vi "GaussianPeakFinder.vi"(3 "Mode":T4, 5 "Traverse line In":T1 {"Carrier_2 Q (l/min)" format="%#.2f"; "Row Duration (mins)" format="%#.1f"; "Row No" min=0; "Trace Gas Concentration (%)" min=0.0 format="%#_4f"; "Carrier_1 Q (l/min)" format="%#.2f"; "Tunnel Speed" format="%#.2f"; "Start X" format="%#.2f"; "Start Y" format="%#.2f"; "Start Z" format="%#.2f"; "End X" format="%#.2f"; "End Y" format="%#.2f"; "End Z" format="%#.2f"; "Averaging time (min)" min=0.0 format="%#.2f"}) -> (0 "Error Message":string, 1 "Status":T5, 2 "Traverse line Out":T1 {"Carrier_2 Q (l/min)" format="%#.2f"; "Row Duration (mins)" format="%#.1f"; "Row No" min=0; "Trace Gas Concentration (%)" min=0.0 format="%#_4f"; "Carrier_1 Q (l/min)" format="%#.2f"; "Tunnel Speed" format="%#.2f"; "Start X" format="%#.2f"; "Start Y" format="%#.2f"; "Start Z" format="%#.2f"; "End X" format="%#.2f"; "End Y" format="%#.2f"; "End Z" format="%#.2f"; "Averaging time (min)" min=0.0 format="%#.2f"})   [LabVIEW 2015]
uses:
  Gen Trav/Traverse_cluster.ctl
  Gen Trav/Spacing.ctl
  Controls/Multi_run_mode.ctl
  Controls/User_Specific_mode.ctl
  Gen Trav/Multi_Run_Status.ctl
  Controls/Setup.ctl
  Controls/Save_Data.ctl
  Utilities/gaussianFit/GaussianGlobal.vi
panel:
  in  "Tab Control":enum32{"GaussianFitGraph", "RunVINamed"}(tab)
  in  "nPointsInRake":i32=3
  out "nPointsSampled":i32
  in  "SpreadFactor":dbl=0.8
  in  "Turbulence":dbl=0.2
  in  "SampleLengthMultiplier":dbl=2.5
  out "MeasurementCenter":sgl
  # "X           Y            Z"
  # "Start"
  # "End"
  # "X           Y            Z"
  # "Start"
  # "End"
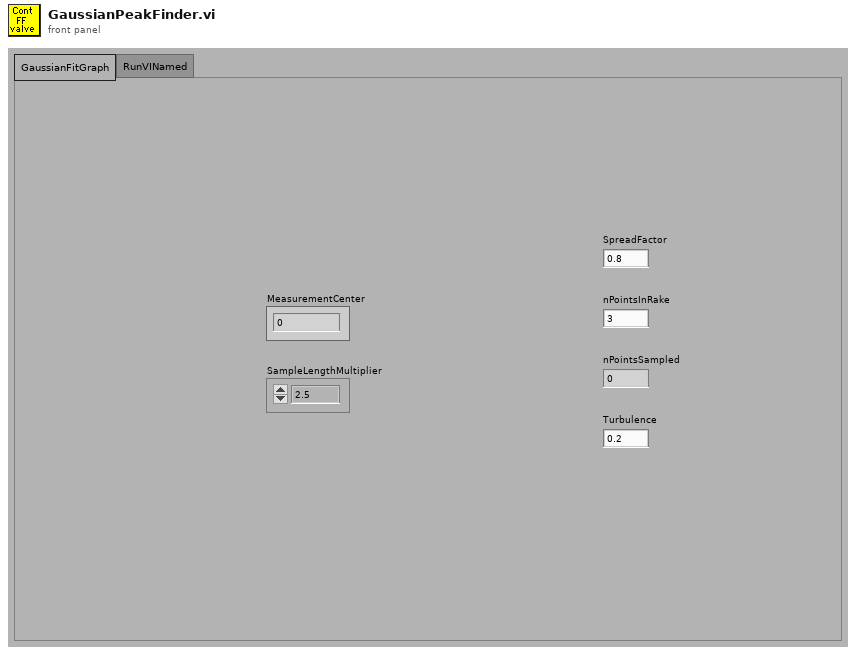
[diagram p1: front panel]
types:
  T1 = typedef "Traverse_cluster.ctl" = cluster{"Start X":sgl, "Start Y":sgl, "Start Z":sgl, "End X":sgl, "End Y":sgl, "End Z":sgl, "No. of pts.":i32, "Spacing":T2, "Filename":path, "Tunnel Speed":dbl, "Averaging time (min)":dbl, "Extra Commands":string, "Carrier_1 Q (l/min)":dbl, "Carrier_2 Q (l/min)":dbl, "Trace Gas Concentration (%)":dbl, "Specific Arguments":string, "Comments":string, "Row No":i32, "Row Type Selector":T3, "Completion time":string, "Row Duration (mins)":dbl, "No. of Valid pts.":i32, "Meas Setup File":string}
  T2 = typedef "Spacing.ctl" = enum16{"Linear", "Log", "Gauss", "Specified", "N/A"}
  T3 = typedef "Multi_run_mode.ctl" = enum16{"Move Traverse Only", "Set Tunnel Speed Only", "Set Source Only", "Set Measurement Conditions", "Single Measurement", "Vertical Profile", "Lateral Profile", "Longitudinal Profile", "Explore Volume", "Multi-Axis Profile", "Auto Calibrate", "Meas Fast FID Bkgnd", "Check Beam Power", "Scanning Valve Measurement", "Run VI Named:", "Set ADAM Ch", "Wait (minutes)", "Send Message", "Synchronize With:", "Fall Back to this Row", "Turn Off Row Repeating", "Blank Row", "Traverse 3D Volume"}
  T4 = typedef "User_Specific_mode.ctl" = enum16{"Check VI only", "Run VI"}
  T5 = typedef "Multi_Run_Status.ctl" = enum16{"Continue", "Jump to Next Point", "Jump to Next Row", "Jump To Fall Back", "Terminate Run"}
  T6 = typedef "Save_Data.ctl" = enum16{"Save No Data", "Save Data"}
  T7 = typedef "Setup.ctl" = enum16{"Run Program", "Show Setup", "Save Current Setup", "Setup Front Panel"}
  T8 = typedef "Status_Cluster.ctl" = cluster{"Status":T5, "Error Type":string, "Error Description":string}
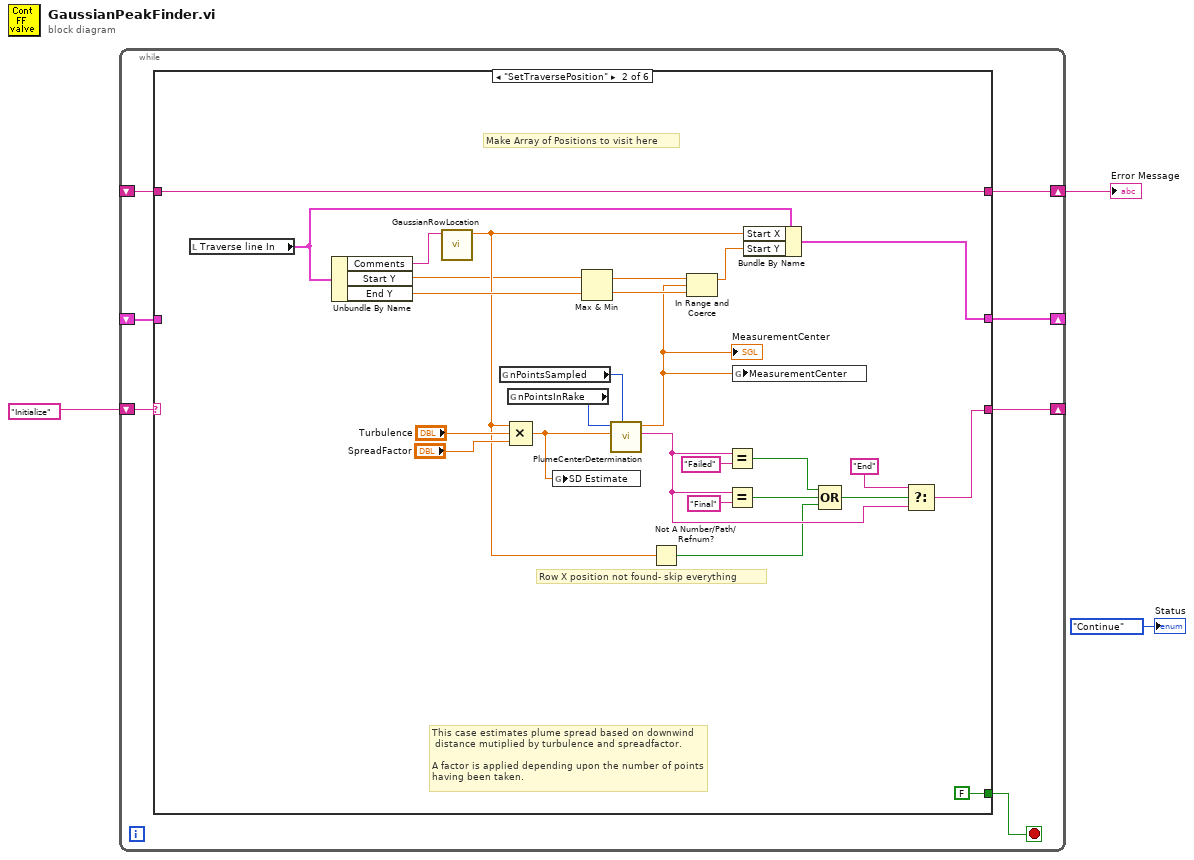
[diagram p0: block diagram]
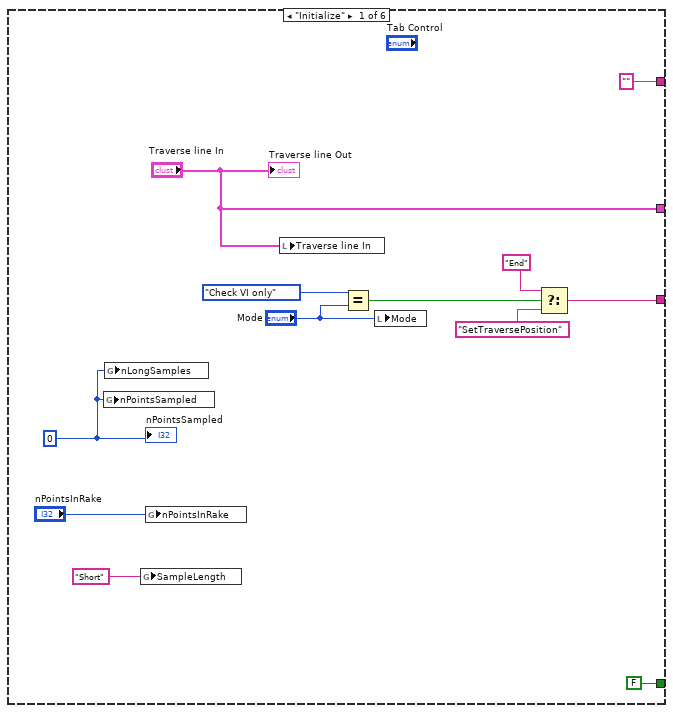
[diagram p2: hidden frame]
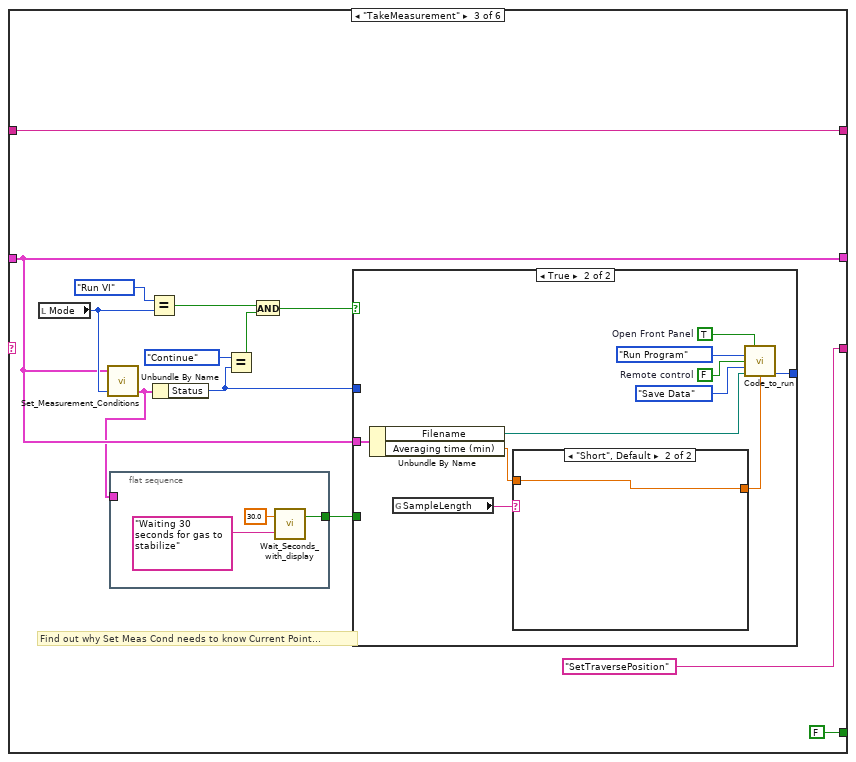
[diagram p3: hidden frame]
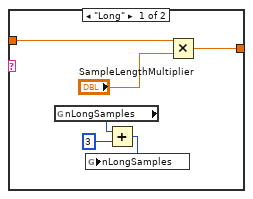
[diagram p5: hidden frame]
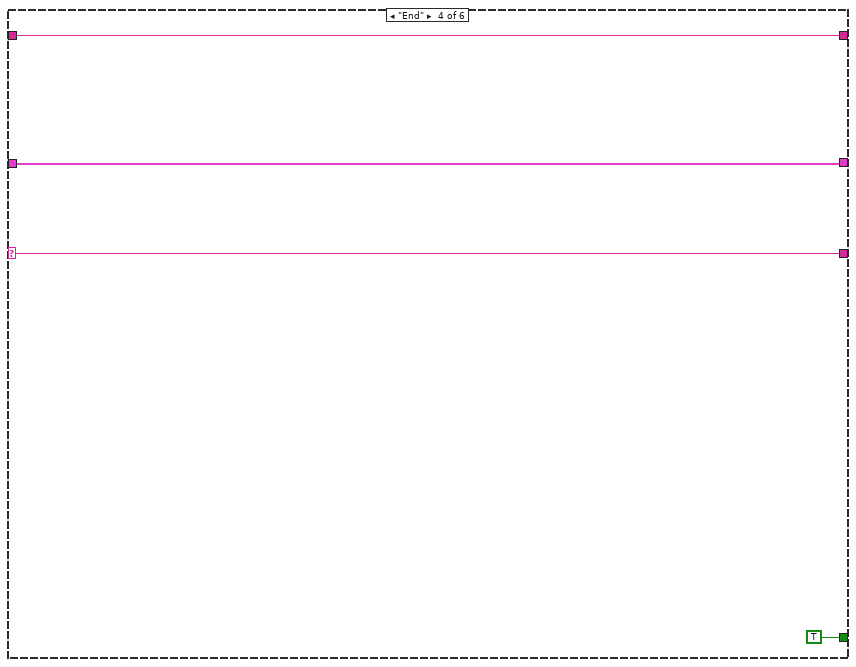
[diagram p6: hidden frame]
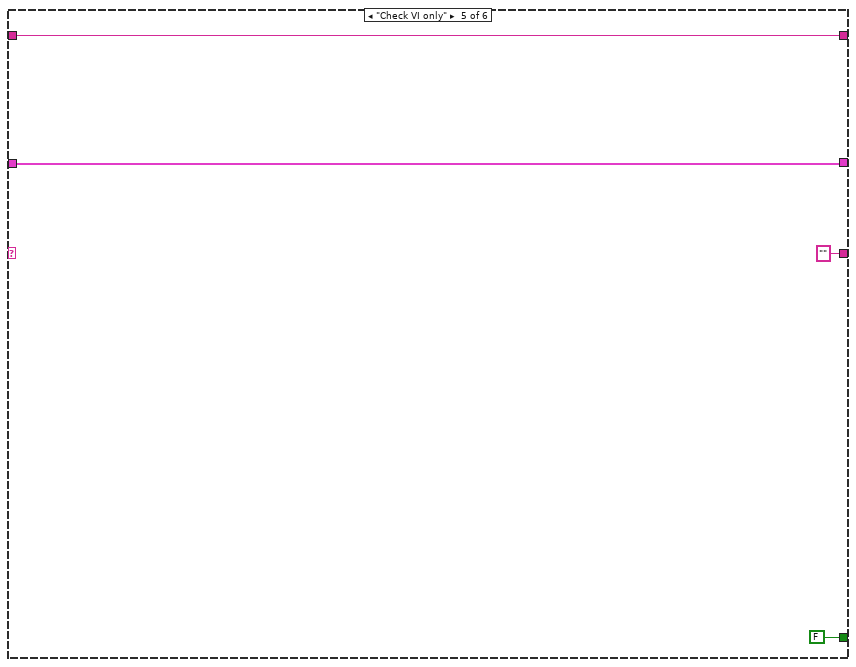
[diagram p7: hidden frame]
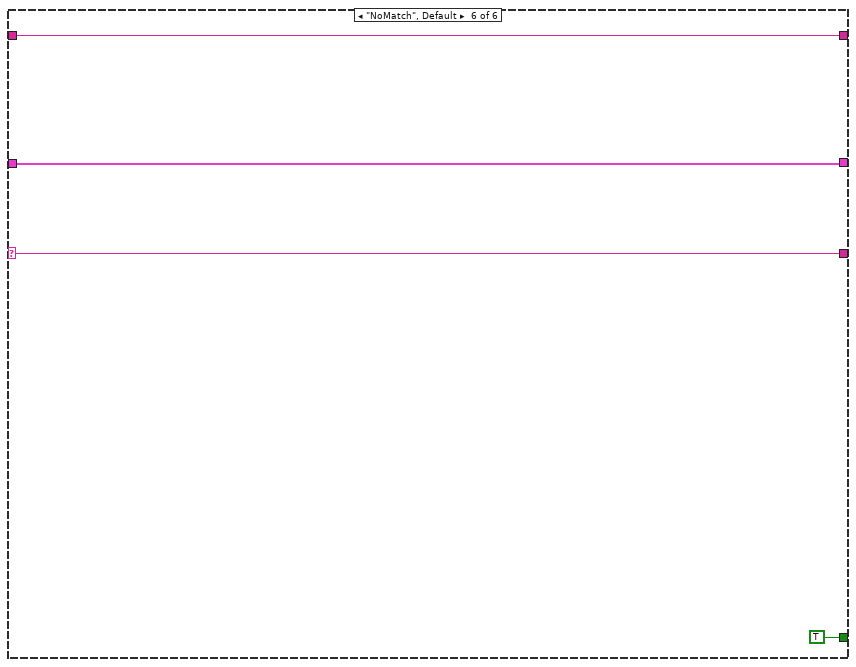
[diagram p8: hidden frame]
diagram:
  n1 = while {
    shift-right: [w8] -> _
    shift-left: _ -> [w7]
    shift-right: [w10] -> w2
    shift-left: _ -> [w5]
    shift-right: [w4] -> _
    shift-left: "Initialize" -> [w9]
    stop <- w6 stop-if-true
    n2 = case shown="\"SetTraversePosition\"" w9 {
      selector: w9 -> [_ _ _ w83 _ w91]
      tunnel: ["" w45 w55 w85 w88 w92] -> w10
      tunnel: ["Traverse line In" w48 w54 w84 w89 w93] -> w8
      tunnel: w7 -> [_ _ w54 w84 w89 w93]
      tunnel: [FALSE FALSE FALSE TRUE FALSE TRUE] -> w6
      tunnel: w5 -> [_ w45 w55 w85 w88 w92]
      tunnel: [w12 w34 "SetTraversePosition" w83 "" w91] -> w4
      frame "Initialize" {
        w18 = 0 ("PointsSampled")
        n3 = global write "GaussianGlobal.vi" "nPointsSampled"(w18) -> ()
        n4 = global write "GaussianGlobal.vi" "nLongSamples"(w18) -> ()
        n5 = global write "GaussianGlobal.vi" "SampleLength"("Short" ("SampleLength")) -> ()
        n6 = global write "GaussianGlobal.vi" "nPointsInRake"("nPointsInRake") -> ()
        n7 = local write "Traverse line In"("Traverse line In") -> ()
        n8 = Equal?(x=User_Specific_mode."Check VI only" ("Mode 2"), y="Mode") -> (x = y?=w15:bool)
        n9 = local write "Mode"("Mode") -> ()
        n10 = Select(t="End", s=w15, f="SetTraversePosition") -> (s? t:f=w12:string)
        "nPointsSampled" <- w18
        "Traverse line Out" <- "Traverse line In"
      }
      frame "SetTraversePosition" {
        # "Row X position not found- skip everything"
        # "This case estimates plume spread based on downwind\n distance mutiplied by turbulence and spreadfactor.\n\nA factor is applied depending upon the number of points\nhaving been taken."
        # "Make Array of Positions to visit here"
        n11 = local read "Traverse line In"() -> (w47:T1)
        n12 = Unbundle By Name(w47) -> ("Comments"=w23:string, "Start Y"=w24:sgl, "End Y"=w44:sgl)
        n13 = call "GaussianRowLocation.vi"("Comments"=w23) -> ("RowXPosition"=w26:dbl)  [unwired: 10 in]
        n14 = global read "GaussianGlobal.vi" "nPointsSampled"() -> (w37:i32)
        n15 = global read "GaussianGlobal.vi" "nPointsInRake"() -> (w38:i32)
        n16 = Compound Arithmetic op=MULTIPLY(w26, "Turbulence", "SpreadFactor") -> (w32:dbl)
        n17 = global write "GaussianGlobal.vi" "SD Estimate"(w32) -> ()
        n18 = Max & Min(x=w24, y=w44) -> (max(x,y)=w43:sgl, min(x,y)=w42:sgl)
        n19 = call "PlumeCenterDetermination.vi"("nPointsSampled"=w37, "SD Estimate"=w32, "nPointsInRake"=w38) -> ("CommandString"=w31:string, "Measurement Center"=w33:sgl)  [unwired: 7 in]
        "MeasurementCenter" <- w33
        n20 = Not A Number/Path/Refnum?(number/path/refnum=w26) -> (NaN/Path/Refnum?=w25:bool)
        n21 = In Range and Coerce(upper limit=w43, x=w33, lower limit=w42) -> (coerced(x)=w41:sgl)  [unwired: 1 out]
        n22 = Equal?(x=w31, y="Failed") -> (x = y?=w29:bool)
        n23 = Equal?(x=w31, y="Final") -> (x = y?=w28:bool)
        n24 = global write "GaussianGlobal.vi" "MeasurementCenter"(w33) -> ()
        n25 = Bundle By Name(cluster=w47, "Start X"=w26, "Start Y"=w41) -> (w48:T1)
        n26 = Compound Arithmetic op=OR(w29, w28, w25) -> (w27:bool)
        n27 = Select(t="End" ("y"), s=w27, f=w31) -> (s? t:f=w34:string)
      }
      frame "TakeMeasurement" {
        # "Find out why Set Meas Cond needs to know Current Point..."
        n28 = local read "Mode"() -> (w57:T4)
        n29 = call "Set_Measurement_Conditions.vi"("Simulate/Run"=w57, "Traverse line"=w54) -> ("Status Cluster"=w49:T8)  [unwired: 3 in]
        n30 = flat-sequence {
          tunnel: [w64] -> w51
          tunnel: w49 -> [_]
          frame #0 {
            n31 = call "Wait_Seconds_with_display.vi"("Message"="Waiting 30 seconds for gas to stabilize", "Seconds to wait"=30.0) -> ("Stopped"=w64:bool)  [unwired: 1 in]
          }
        }
        n32 = Equal?(x=User_Specific_mode."Run VI" ("Mode"), y=w57) -> (x = y?=w61:bool)
        n33 = Unbundle By Name(w49) -> ("Status"=w52:T5)
        n34 = Equal?(x=Multi_Run_Status."Continue" ("Status"), y=w52) -> (x = y?=w58:bool)
        n35 = And(x=w61, y=w58) -> (x .and. y?=w50:bool)
        n36 = case shown="True" w50 {
          tunnel: w54 -> [_ w75]
          tunnel: w52 -> [w65 _]
          tunnel: [w65 w70] -> _
          tunnel: w51 -> [_ _]
          frame False {
          }
          frame True {
            w73 = TRUE  # Open Front Panel
            w74 = FALSE  # Remote control
            n37 = Unbundle By Name(w75) -> ("Filename"=w69:path, "Averaging time (min)"=w67:dbl)
            n38 = global read "GaussianGlobal.vi" "SampleLength"() -> (w68:string)
            n39 = case shown="\"Short\", Default" w68 {
              tunnel: w67 -> [w81 w82]
              tunnel: [w79 w82] -> w66
              frame "Long" {
                n40 = global read "GaussianGlobal.vi" "nLongSamples"() -> (w76:i32)
                n41 = Add(x=w76, y=3) -> (x+y=w77:i32)
                n42 = global write "GaussianGlobal.vi" "nLongSamples"(w77) -> ()
                n43 = Multiply(x=w81, y="SampleLengthMultiplier") -> (x*y=w79:dbl)
              }
              frame "Short", Default {
              }
            }
            n44 = call "Code_to_run.vi"("Open Front Panel"=w73, "setup"=Setup."Run Program", "Remote control"=w74, "File"=Save_Data."Save Data", "Results Filename"=w69, "Averaging time (min)"=w66) -> ("Status"=w70:T5)  [unwired: 9 in]
          }
        }
      }
      frame "End" {
      }
      frame "Check VI only" {
      }
      frame "NoMatch", Default {
      }
    }
  }
  "Error Message" <- w2
  "Status" <- Multi_Run_Status."Continue" ("Status")
